vi "Event-Driven Scenario (Polling Method).vi"() -> ()   [LabVIEW 2014]
panel:
  out "波形图":dynamicdata(graph)
  in  "采集数据":bool
  out "温度（华氏度）":dbl=32.0
  in  "温度（摄氏度）":dbl
  in  "时间检查":bool
  out "当前时间":timestamp
  in  "停止":bool
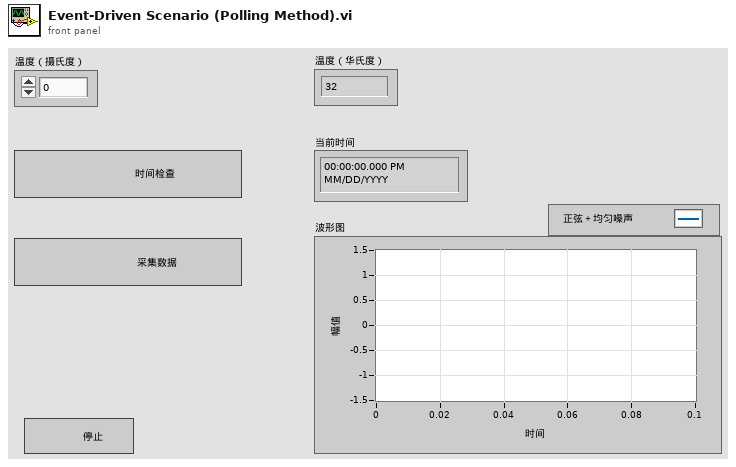
[diagram p1: front panel]
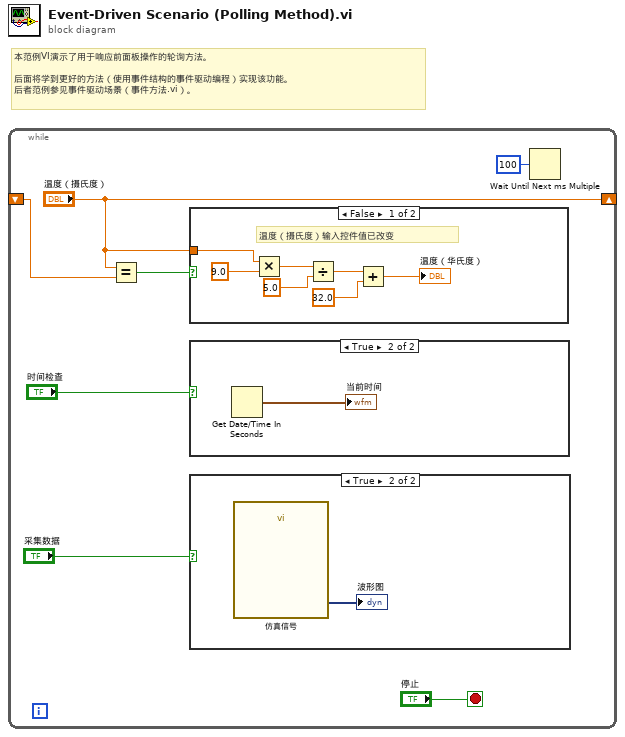
[diagram p0: block diagram]
diagram:
  # "本范例VI演示了用于响应前面板操作的轮询方法。\n\n后面将学到更好的方法（使用事件结构的事件驱动编程）实现该功能。\n后者范例参见事件驱动场景（事件方法.vi）。"
  n1 = while {
    shift-right: ["温度（摄氏度）"] -> _
    shift-left: _ -> [w4]
    stop <- "停止" stop-if-true
    n2 = Equal?(x="温度（摄氏度）", y=w4) -> (x = y?=w3:bool)
    n3 = case shown="False" w3 {
      tunnel: "温度（摄氏度）" -> [w8 _]
      frame False {
        # "温度（摄氏度）输入控件值已改变"
        n4 = Multiply(x=w8, y=9.0) -> (x*y=w13:dbl)
        n5 = Divide(x=w13, y=5.0) -> (x/y=w11:dbl)
        n6 = Add(x=w11, y=32.0) -> (x+y=→"温度（华氏度）":dbl)
      }
      frame True {
      }
    }
    n7 = case shown="True" "时间检查" {
      frame False {
      }
      frame True {
        n8 = Get Date/Time In Seconds() -> (seconds since 1Jan1904=→"当前时间":timestamp)
      }
    }
    n9 = case shown="True" "采集数据" {
      frame False {
      }
      frame True {
        n10 = call "仿真信号"() -> ("Sine with Uniform Noise"=→"波形图":dynamicdata)  [unwired: 14 in, 1 out]
      }
    }
    n11 = Wait Until Next ms Multiple(millisecond multiple=u32 100 ("毫秒倍数")) -> ()  [unwired: 1 out]
  }
